vi "doubleArrayToStringWithBrackets.vi"(8 "error in (no error)":errorcluster, 10 "presicion (0)":u8, 11 "value":dbl[](array[numeric])) -> (0 "error out":errorcluster, 3 "String":string)   [LabVIEW 2018]
doc: "Convert a double array of 1-dimension to a table in string form separated by comma and between brackets."
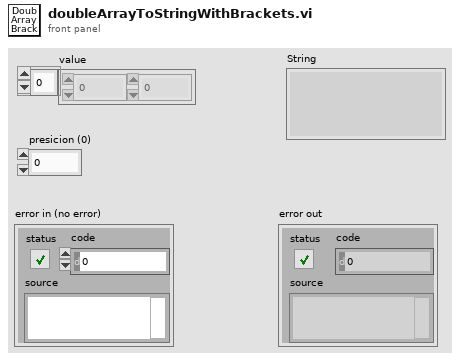
[diagram p1: front panel]
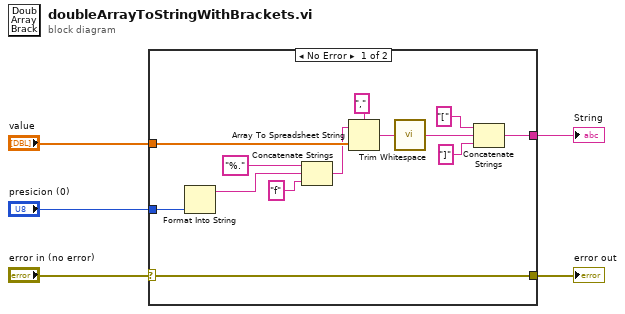
[diagram p0: block diagram]
diagram:
  n1 = case shown="No Error" "error in (no error)" {
    selector: "error in (no error)" -> [w6 w19]
    tunnel: [w18 _] -> w5
    tunnel: "presicion (0)" -> [w17 _]
    tunnel: "value" -> [w16 _]
    tunnel: [w6 w19] -> w1
    frame No Error {
      n2 = Format Into String(w17) -> (resulting string=w9:string)  [unwired: 3 in, 1 out]
      n3 = Concatenate Strings("%." ("format string"), w9, "f" ("format string")) -> (w14:string)
      n4 = Array To Spreadsheet String(delimiter (Tab)=",", array=w16, 3:w14) -> (spreadsheet string=w11:string)
      n5 = call <vilib>:"Trim Whitespace.vi"("string"=w11) -> ("trimmed string"=w15:string)  [unwired: 1 in]
      n6 = Concatenate Strings("[" ("string"), w15, "]" ("string")) -> (w18:string)
    }
    frame Error {
    }
  }
  "String" <- w5
  "error out" <- w1
